vi "R5Initialize.vi"(8 "error in (no error)":errorcluster) -> (0 "error out":errorcluster)   [LabVIEW 2016]
uses:
  Controls/pH_SetParams Standard.ctl
  R5Controls/R5SBR_SetParams.ctl
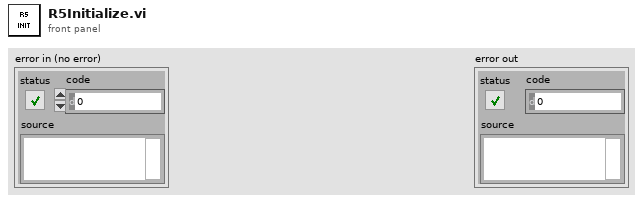
[diagram p1: front panel]
types:
  T1 = cluster{"Set Point, mg/L":dbl, "Tolerance, mg/L":dbl, "N2 Valve Gain":dbl, "Air Valve Gain":dbl, "DO Cycle, min":dbl, "DO Fraction":dbl}
  T2 = typedef "R5SBR_SetParams.ctl" = cluster{"Phase":string, "Time, min":dbl, "SBR_Manual":cluster{"Influent Pump":bool, "Effluent Pump":bool}}[]
  T3 = typedef "pH_SetParams Standard.ctl" = cluster{"Set Point":dbl, "Tolerance":dbl, "Pump Time On, secs":dbl}
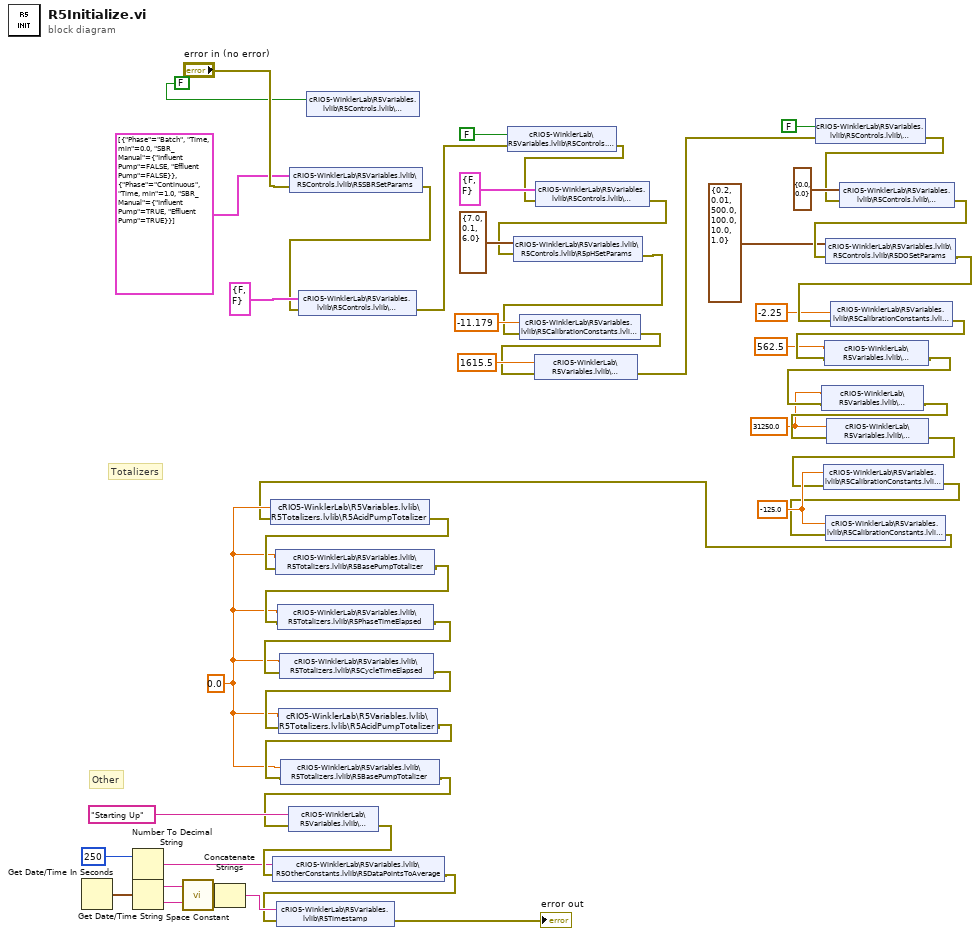
[diagram p0: block diagram]
diagram:
  w13 = 0.0 ("R1PhaseTimeElapsed")
  w22 = 31250.0 ("R1AirSlope")
  w21 = -125.0 ("R1N2Intercept")
  # "Totalizers"
  # "Other"
  n1 = Get Date/Time In Seconds() -> (seconds since 1Jan1904=w49:timestamp)
  n2 = Number To Decimal String(number=250 ("R1DataPointsToAverage")) -> (decimal integer string=w9:string)  [unwired: 1 in]
  n3 = Get Date/Time String(seconds (now)=w49) -> (date string=w46:string, time string=w48:string)  [unwired: 2 in]
  n4 = call <vilib>:"Space Constant.vi"() -> ("String"=w47:string)
  n5 = Concatenate Strings(w46, w47, w48) -> (w8:string)
  n6 = shared-variable "cRIO5-WinklerLab\\R5Variables.lvlib\\R5Controls.lvlib\\R5SBRSetParams"(T2 [{"Phase"="Batch", "Time, min"=0.0, "SBR_Manual"={"Influent Pump"=FALSE, "Effluent Pump"=FALSE}}, {"Phase"="Continuous", "Time, min"=1.0, "SBR_Manual"={"Influent Pump"=TRUE, "Effluent Pump"=TRUE}}] ("R5SBRSetParams"), error in="error in (no error)") -> (error out=w44:errorcluster)
  n7 = shared-variable "cRIO5-WinklerLab\\R5Variables.lvlib\\R5Controls.lvlib\\R5SBRManual"(cluster{"Media Pump":bool, "Effluent Pump":bool} {"Media Pump"=FALSE, "Effluent Pump"=FALSE} ("R5SBRManual"), error in=w44) -> (error out=w31:errorcluster)
  n8 = shared-variable "cRIO5-WinklerLab\\R5Variables.lvlib\\R5Controls.lvlib\\R5SBRSwitch"(FALSE ("R1SBRSwitch")) -> ()  [unwired: 1 in, 1 out]
  n9 = shared-variable "cRIO5-WinklerLab\\R5Variables.lvlib\\R5Controls.lvlib\\R5pHSwitch"(FALSE ("R1pHSwitch"), error in=w31) -> (error out=w33:errorcluster)
  n10 = shared-variable "cRIO5-WinklerLab\\R5Variables.lvlib\\R5Controls.lvlib\\R5pHManual"(cluster{"Acid Pump":bool, "Base Pump":bool} {"Acid Pump"=FALSE, "Base Pump"=FALSE} ("R1pHManual"), error in=w33) -> (error out=w35:errorcluster)
  n11 = shared-variable "cRIO5-WinklerLab\\R5Variables.lvlib\\R5Controls.lvlib\\R5pHSetParams"(T3 {"Set Point"=7.0, "Tolerance"=0.1, "Pump Time On, secs"=6.0} ("R1pHSetParams"), error in=w35) -> (error out=w36:errorcluster)
  n12 = shared-variable "cRIO5-WinklerLab\\R5Variables.lvlib\\R5CalibrationConstants.lvlib\\R5pHIntercept"(-11.179 ("R12pHInt"), error in=w36) -> (error out=w39:errorcluster)
  n13 = shared-variable "cRIO5-WinklerLab\\R5Variables.lvlib\\R5CalibrationConstants.lvlib\\R5pHSlope"(1615.5 ("R1pHSlope"), error in=w39) -> (error out=w3:errorcluster)
  n14 = shared-variable "cRIO5-WinklerLab\\R5Variables.lvlib\\R5Controls.lvlib\\R5DOSwitch"(FALSE ("R1pHSwitch"), error in=w3) -> (error out=w2:errorcluster)
  n15 = shared-variable "cRIO5-WinklerLab\\R5Variables.lvlib\\R5Controls.lvlib\\R5DOManual"(cluster{"Air MFC":dbl, "N2 MFC":dbl} {"Air MFC"=0.0, "N2 MFC"=0.0} ("R1DOManual"), error in=w2) -> (error out=w29:errorcluster)
  n16 = shared-variable "cRIO5-WinklerLab\\R5Variables.lvlib\\R5Controls.lvlib\\R5DOSetParams"(T1 {"Set Point, mg/L"=0.2, "Tolerance, mg/L"=0.01, "N2 Valve Gain"=500.0, "Air Valve Gain"=100.0, "DO Cycle, min"=10.0, "DO Fraction"=1.0} ("R5DOSetParams"), error in=w29) -> (error out=w28:errorcluster)
  n17 = shared-variable "cRIO5-WinklerLab\\R5Variables.lvlib\\R5CalibrationConstants.lvlib\\R5DOIntercept"(-2.25 ("R1DOInt"), error in=w28) -> (error out=w26:errorcluster)
  n18 = shared-variable "cRIO5-WinklerLab\\R5Variables.lvlib\\R5CalibrationConstants.lvlib\\R5DOSlope"(562.5 ("R1DOSlope"), error in=w26) -> (error out=w24:errorcluster)
  n19 = shared-variable "cRIO5-WinklerLab\\R5Variables.lvlib\\R5CalibrationConstants.lvlib\\R5N2Slope"(w22, error in=w24) -> (error out=w23:errorcluster)
  n20 = shared-variable "cRIO5-WinklerLab\\R5Variables.lvlib\\R5CalibrationConstants.lvlib\\R5AirSlope"(w22, error in=w23) -> (error out=w20:errorcluster)
  n21 = shared-variable "cRIO5-WinklerLab\\R5Variables.lvlib\\R5CalibrationConstants.lvlib\\R5AirIntercept"(w21, error in=w20) -> (error out=w19:errorcluster)
  n22 = shared-variable "cRIO5-WinklerLab\\R5Variables.lvlib\\R5CalibrationConstants.lvlib\\R5N2Intercept"(w21, error in=w19) -> (error out=w5:errorcluster)
  n23 = shared-variable "cRIO5-WinklerLab\\R5Variables.lvlib\\R5Totalizers.lvlib\\R5AcidPumpTotalizer"(w13, error in=w5) -> (error out=w18:errorcluster)
  n24 = shared-variable "cRIO5-WinklerLab\\R5Variables.lvlib\\R5Totalizers.lvlib\\R5BasePumpTotalizer"(w13, error in=w18) -> (error out=w17:errorcluster)
  n25 = shared-variable "cRIO5-WinklerLab\\R5Variables.lvlib\\R5Totalizers.lvlib\\R5PhaseTimeElapsed"(w13, error in=w17) -> (error out=w16:errorcluster)
  n26 = shared-variable "cRIO5-WinklerLab\\R5Variables.lvlib\\R5Totalizers.lvlib\\R5CycleTimeElapsed"(w13, error in=w16) -> (error out=w15:errorcluster)
  n27 = shared-variable "cRIO5-WinklerLab\\R5Variables.lvlib\\R5Totalizers.lvlib\\R5AcidPumpTotalizer"(w13, error in=w15) -> (error out=w14:errorcluster)
  n28 = shared-variable "cRIO5-WinklerLab\\R5Variables.lvlib\\R5Totalizers.lvlib\\R5BasePumpTotalizer"(w13, error in=w14) -> (error out=w11:errorcluster)
  n29 = shared-variable "cRIO5-WinklerLab\\R5Variables.lvlib\\R5Status"("Starting Up" ("R1Status"), error in=w11) -> (error out=w10:errorcluster)
  n30 = shared-variable "cRIO5-WinklerLab\\R5Variables.lvlib\\R5OtherConstants.lvlib\\R5DataPointsToAverage"(w9, error in=w10) -> (error out=w7:errorcluster)
  n31 = shared-variable "cRIO5-WinklerLab\\R5Variables.lvlib\\R5Timestamp"(w8, error in=w7) -> (error out=→"error out":errorcluster)
